vi "Obtain Control Cluster.vi"(9 "I/O":bool=TRUE, 10 "Dispense":bool=TRUE, 11 "Motion":bool=TRUE) -> (3 "Control Out":T1={"I-O.lvclass"=refnum, "Gantry"=refnum, "Dispenser"="COM1"})   [LabVIEW 2020, in "Controller.lvclass"]
uses:
  Controller.lvclass
  I-O/NI-DAQ/NI-DAQ.lvclass
  Drivers/Aerotech A3200/Aerotech.lvlib
  Drivers/EFD Ultimus V/EFD Ultimus V.lvlib
  I-O/I-O.lvclass
  Controllers.ctl
  C:/Program Files (x86)/Aerotech/A3200/LabVIEW/2010/Bin/Aerotech.A3200.dll
  Program Files (x86)/Aerotech/A3200/LabVIEW/2010/Bin/Aerotech.A3200.dll
panel:
  in  "Control":T1={"I-O.lvclass"=refnum, "Gantry"=refnum, "Dispenser"="COM1"}
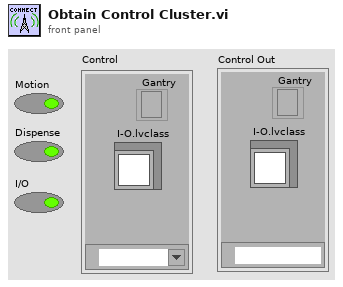
[diagram p1: front panel]
types:
  T1 = typedef "Controller.lvclass/Controllers.ctl" = cluster{"I-O.lvclass":refnum<class "I-O.lvclass">, "Gantry":refnum<k24>, "Dispenser":refnum<visa-resource-name>}
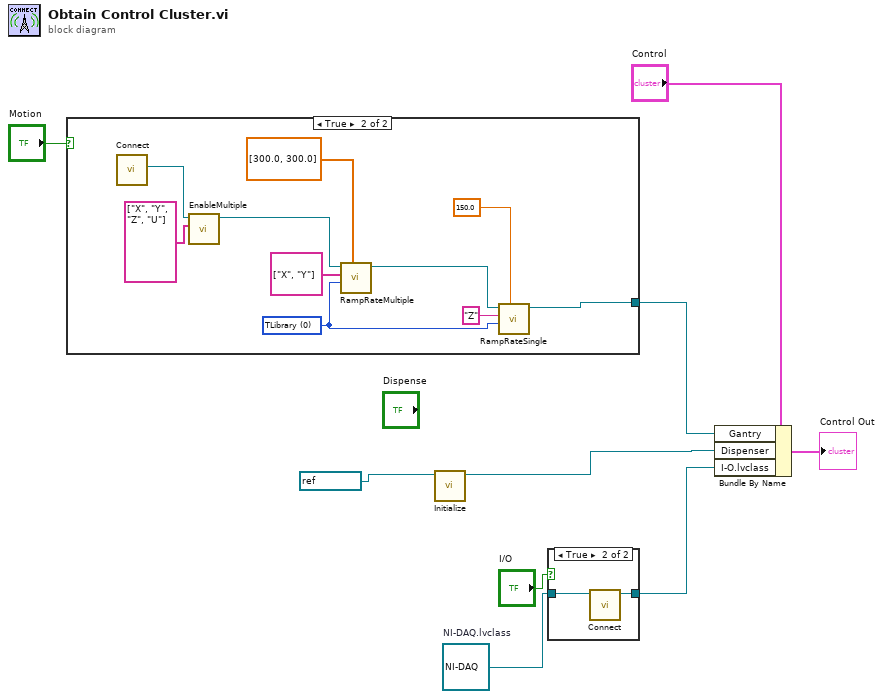
[diagram p0: block diagram]
diagram:
  w5 = refnum<class "NI-DAQ.lvclass"> refnum  # NI-DAQ.lvclass
  n1 = case shown="True" "Motion" {
    tunnel: [_ w11] -> w3
    frame False {
    }
    frame True {
      w12 = 0 items=["TLibrary", "T01", "T02", "T03", "T04", "T05", "T06", "T07", "T08", "T09", "T10", "T11", "T12", "T13", "T14", "T15", "T16", "T17", "T18", "T19", "T20", "T21", "T22", "T23", "T24", "T25", "T26", "T27", "T28", "T29", "T30", "T31"] ("task id")
      n2 = call "Connect.vi"() -> ("controller"=w19:refnum<k24>)  [unwired: 10 in, 1 out]
      n3 = call "EnableMultiple.vi"("axis names"=string[] ["X", "Y", "Z", "U"], "controller in"=w19) -> ("controller out"=w17:refnum<k24>)  [unwired: 8 in, 1 out]
      n4 = call "RampRateMultiple.vi"("ramp rates"=dbl[] [300.0, 300.0], "task id"=w12, "axis names"=string[] ["X", "Y"], "controller in"=w17) -> ("controller out"=w14:refnum<k24>)  [unwired: 6 in, 1 out]
      n5 = call "RampRateSingle.vi"("ramp rate"=150.0, "task id"=w12, "axis name"="Z", "controller in"=w14) -> ("controller out"=w11:refnum<k24>)  [unwired: 6 in, 1 out]
    }
  }
  n6 = call "Initialize.vi"("VISA resource name"=refnum<visa-resource-name> "COM4" ("Dispenser")) -> ("VISA resource name out"=w1:refnum<visa-resource-name>)  [unwired: 9 in, 1 out]
  n7 = case shown="True" "I/O" {
    tunnel: w5 -> [w20 w22]
    tunnel: [w20 w21] -> w7
    frame False {
    }
    frame True {
      n8 = call-dynamic "Connect.vi"("NI-DAQ in"=w22) -> ("NI-DAQ out"=w21:refnum<class "NI-DAQ.lvclass">)  [unwired: 9 in, 1 out]
    }
  }
  n9 = Bundle By Name(cluster="Control", "Gantry"=w3, "Dispenser"=w1, "I-O.lvclass"=w7) -> (→"Control Out":T1)
